vi "get_autostart_flag.vi"(8 "error in (no error)":errorcluster, 11 "GenericScanMode in":refnum<class "GenericImagingMode.lvclass">) -> (0 "error out":errorcluster, 2 "autostart?":bool, 3 "GenericScanMode out":refnum<class "GenericImagingMode.lvclass">)   [LabVIEW 2010, in "GenericImagingMode.lvclass"]
uses:
  GenericImagingMode.lvclass
  GenericImagingMode.lvclass/GenericImagingMode.ctl
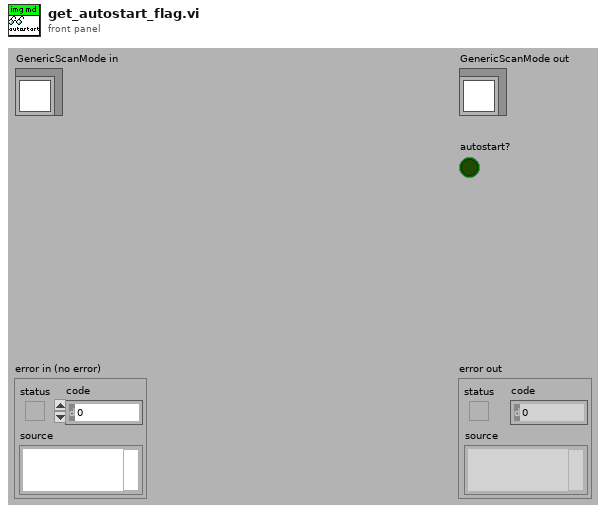
[diagram p1: front panel]
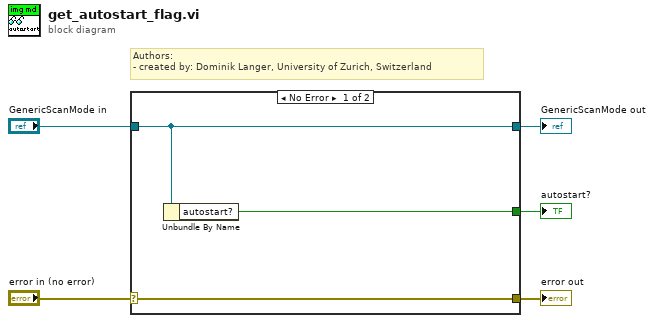
[diagram p0: block diagram]
diagram:
  # "Authors: \n- created by: Dominik Langer, University of Zurich, Switzerland"
  n1 = case shown="No Error" "error in (no error)" {
    selector: "error in (no error)" -> [w8 w9]
    tunnel: [w8 w9] -> w4
    tunnel: [w7 w10] -> w2
    tunnel: "GenericScanMode in" -> [w7 w10]
    tunnel: [w6 _] -> w1
    frame No Error {
      n2 = Unbundle By Name(w7) -> ("autostart?"=w6:bool)
    }
    frame Error {
    }
  }
  "error out" <- w4
  "GenericScanMode out" <- w2
  "autostart?" <- w1
